vi "ProdaNG.Configurator.Popup.Add.vi"(6 "units simple":T1[](array[typedef]), 10 "Selected element":T2) -> (1 "Selected elements value out":T4, 2 "Selected element out":T2, 4 "Reason out":string, 5 "OK?":bool)   [LabVIEW 2016]
uses:
  ProdaNG.Tree.Fglb.Data.ctl
  ProdaNG.Tree.Fglb.Element.ctl
  ProdaNG.Tree.Fglb.Value.ctl
  Controls/ProdaNG.UnitSimple.ctl
panel:
  in  "Unit":i32(ring) items=["%"=1, "A"=12, "ASCII"=20, "Hz"=16, "N"=11, "Nm"=21, "V"=13, "angle"=17, "bar"=2, "bar (abs)"=3, "bar/s"=5, "bool"=19, "ccm/min"=24, "count"=18, "digit"=26, "kg"=22, "kohm"=15, "l/min"=7, "mA"=25, "mA/s"=30, "mBar/s"=29, "mbar"=4, "mbar/s"=6, "mm"=10, "ms"=9, "obr/min"=23, "ohm"=14, "s"=8, "stC"=28, "unknown"=-1, "us"=27]
  in  "Type":T5(ring)
  in  "Value2":dbl caption="High Limit" format="%.3f"
  in  "Value1":dbl caption="Low Limit / Param Value" format="%.3f"
  in  "Order":i32=1 min=1
  in  "Reason":string
  in  "Description":string
  in  "Button.Cancel":bool
  in  "Button.OK":bool
  out "Msg":string
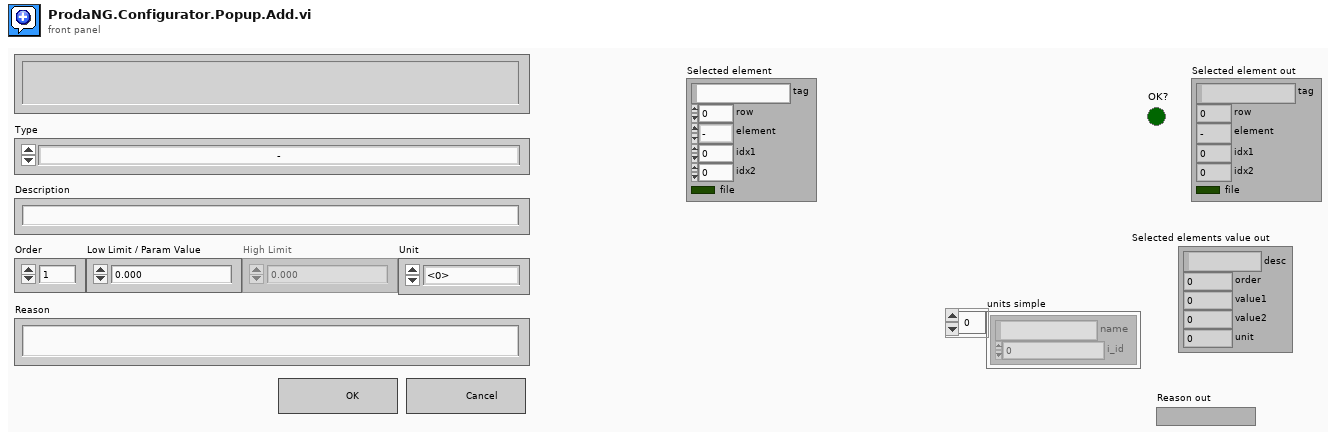
[diagram p1: front panel]
types:
  T1 = typedef "ProdaNG.UnitSimple.ctl" = cluster{"name":string, "i_id":i32}
  T2 = typedef "ProdaNG.Tree.Fglb.Data.ctl" = cluster{"tag":string, "row":i32, "element":T3, "idx1":i32, "idx2":i32, "file":bool}
  T3 = typedef "ProdaNG.Tree.Fglb.Element.ctl" = enum16{"-", "PP", "TS", "TP", "TV"}
  T4 = typedef "ProdaNG.Tree.Fglb.Value.ctl" = cluster{"desc":string, "order":i32, "value1":dbl, "value2":dbl, "unit":i32}
  T5 = enum16{"-", "Process Parameter", "Test Step", "Test Parameter", "Test Value"}
  T6 = enum8{"Enabled", "Disabled", "Disabled and Grayed Out"}
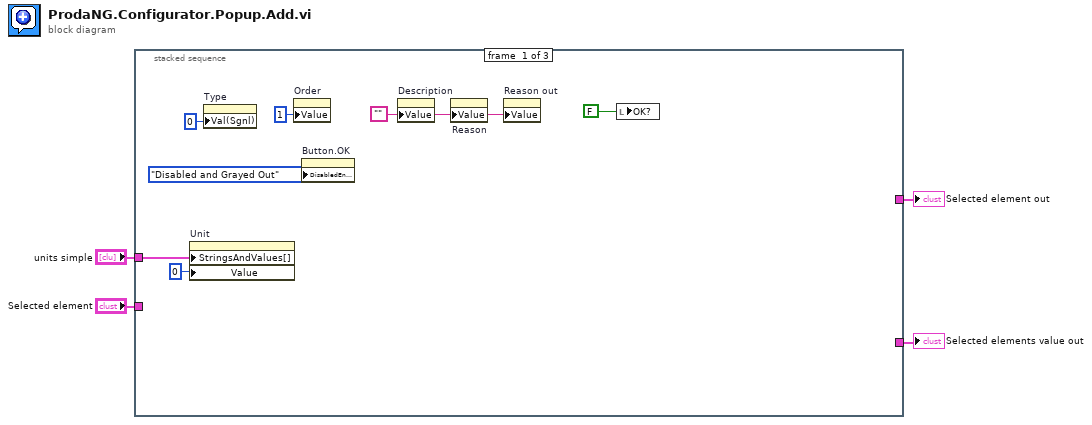
[diagram p0: block diagram]
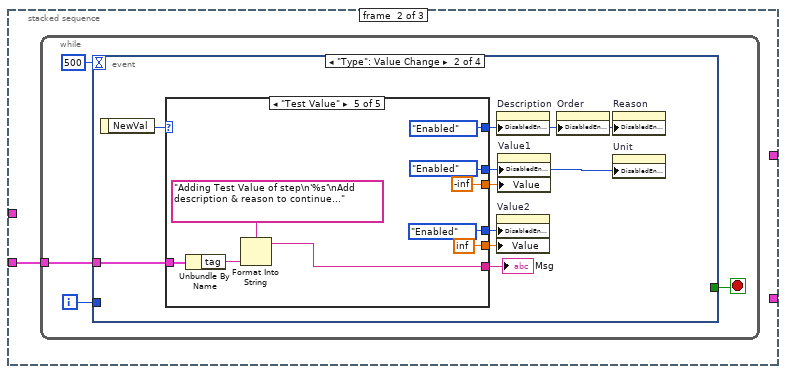
[diagram p2: hidden frame]
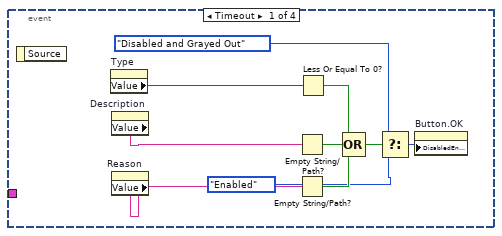
[diagram p3: hidden frame]
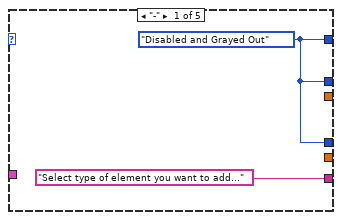
[diagram p4: hidden frame]
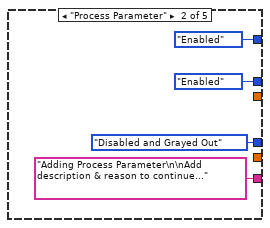
[diagram p5: hidden frame]
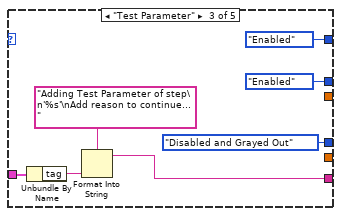
[diagram p6: hidden frame]
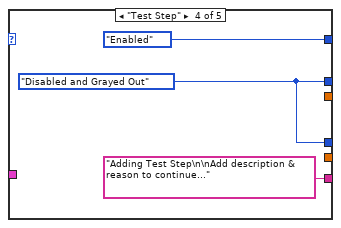
[diagram p7: hidden frame]
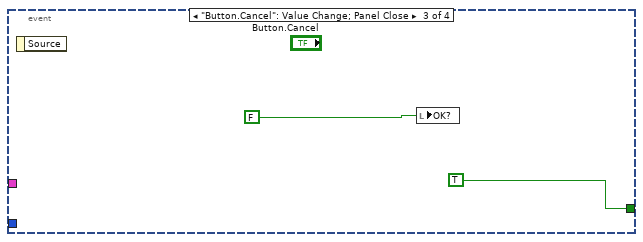
[diagram p8: hidden frame]
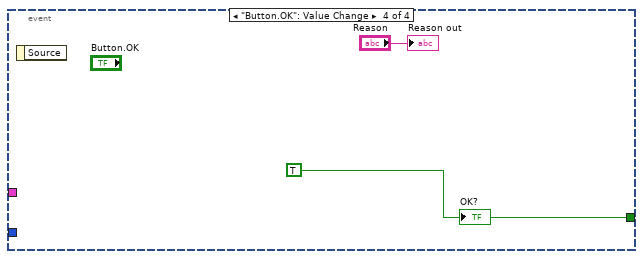
[diagram p9: hidden frame]
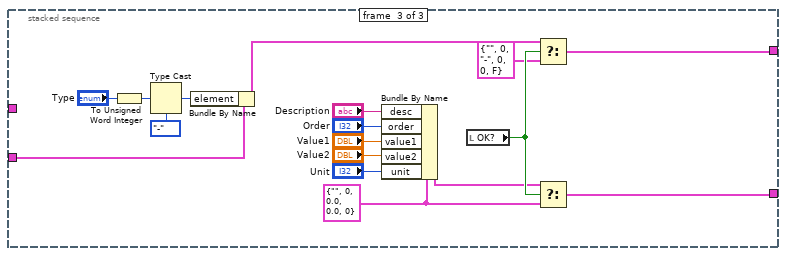
[diagram p10: hidden frame]
diagram:
  n1 = stacked-sequence {
    tunnel: [_ _ w80] -> w4
    tunnel: "Selected element" -> [_ w12 w78]
    tunnel: [_ _ w75] -> w2
    tunnel: "units simple" -> [w7 _ _]
    frame #0 {
      w9 = ""
      n2 = property on="Unit" class="Ring (strict)"("StringsAndValues[]"=w7, "Value"=0) -> ()  [unwired: 2 in, 2 out]
      n3 = property on="Type" class="Enum (strict)"("Val(Sgnl)"=0) -> ()  [unwired: 2 in, 2 out]
      n4 = property on="Order" class="DigNum (strict)"("Value"=1 ("Order")) -> ()  [unwired: 2 in, 2 out]
      n5 = property on="Button.OK" class="Bool"("DisabledEnum"=T6."Disabled and Grayed Out" ("Disabled")) -> ()  [unwired: 2 in, 2 out]
      n6 = property on="Description" class="Str"("Value"=w9) -> ()  [unwired: 2 in, 2 out]
      n7 = property on="Reason" class="Str"("Value"=w9) -> ()  [unwired: 2 in, 2 out]
      n8 = property on="Reason out" class="Str"("Value"=w9) -> ()  [unwired: 2 in, 2 out]
      n9 = local write "OK?"(FALSE ("OK?")) -> ()
    }
    frame #1 {
      n10 = while {
        tunnel: w12 -> [w13]
        i -> [w14]
        stop <- w16 stop-if-true
        n11 = event shown="[1] \"Type\": Value Change" {
          selector: _ -> [_ _ _ _]
          dyn-events: _ -> [_ _ _ _]
          timeout: 500 -> [_ _ _ _]
          tunnel: [_ _ TRUE ("OK?") w63] -> w16
          tunnel: w14 -> [_ _ _ _]
          tunnel: w13 -> [_ w29 _ _]
          event Timeout {
            n12 = event-data() -> ()  [unwired: 1 in, 1 out]
            n13 = property on="Type" class="Enum (strict)"() -> ("Value"=w22:T5)  [unwired: 2 in, 2 out]
            n14 = property on="Description" class="Str"() -> ("Value"=w20:string)  [unwired: 2 in, 2 out]
            n15 = property on="Reason" class="Str"() -> ("Value"=w21:string)  [unwired: 2 in, 2 out]
            n16 = Empty String/Path?(string/path=w20) -> (empty?=w23:bool)
            n17 = Empty String/Path?(string/path=w21) -> (empty?=w24:bool)
            n18 = Less Or Equal To 0?(x=w22) -> (x <= 0?=w25:bool)
            n19 = Compound Arithmetic op=OR(w25, w23, w24) -> (w26:bool)
            n20 = Select(t=T6."Disabled and Grayed Out" ("Disabled"), s=w26, f=T6."Enabled" ("Disabled")) -> (s? t:f=w17:T6)
            n21 = property on="Button.OK" class="Bool"("DisabledEnum"=w17) -> ()  [unwired: 2 in, 2 out]
          }
          event "Type": Value Change {
            n22 = event-data() -> ("NewVal"=w34:T5)  [unwired: 1 in]
            n23 = case shown="\"Test Value\"" w34 {
              tunnel: [w35 T6."Enabled" ("Disabled") T6."Enabled" ("Disabled") T6."Enabled" ("Disabled") T6."Enabled" ("Disabled")] -> w33
              tunnel: [w35 T6."Enabled" ("Disabled") T6."Enabled" ("Disabled") w49 T6."Enabled" ("Disabled")] -> w30
              tunnel: [_ _ _ _ -inf] -> w32
              tunnel: [_ _ _ _ inf] -> w31
              tunnel: w29 -> [_ _ w42 _ w54]
              tunnel: ["Select type of element you want to add..." ("format string") "Adding Process Parameter\n\nAdd description & reason to continue..." ("format string") w41 "Adding Test Step\n\nAdd description & reason to continue..." ("format string") w51] -> w28
              tunnel: [w35 T6."Disabled and Grayed Out" ("Disabled") T6."Disabled and Grayed Out" ("Disabled") w49 T6."Enabled" ("Disabled")] -> w27
              frame "-" {
                w35 = T6."Disabled and Grayed Out" ("Disabled")
              }
              frame "Process Parameter" {
              }
              frame "Test Parameter" {
                n24 = Unbundle By Name(w42) -> ("tag"=w44:string)
                n25 = Format Into String(format string="Adding Test Parameter of step\n'%s'\nAdd reason to continue...", w44) -> (resulting string=w41:string)  [unwired: 2 in, 1 out]
              }
              frame "Test Step" {
                w49 = T6."Disabled and Grayed Out" ("Disabled")
              }
              frame "Test Value" {
                n26 = Unbundle By Name(w54) -> ("tag"=w53:string)
                n27 = Format Into String(format string="Adding Test Value of step\n'%s'\nAdd description & reason to continue...", w53) -> (resulting string=w51:string)  [unwired: 2 in, 1 out]
              }
            }
            "Msg" <- w28
            n28 = property on="Description" class="Str"("DisabledEnum"=w33) -> ()  [unwired: 2 in, 2 out]
            n29 = property on="Value2" class="DigNum (strict)"("DisabledEnum"=w27, "Value"=w31) -> ()  [unwired: 2 in, 2 out]
            n30 = property on="Value1" class="DigNum (strict)"("DisabledEnum"=w30, "Value"=w32) -> ()  [unwired: 2 in, 2 out]
            n31 = property on="Order" class="DigNum (strict)"("DisabledEnum"=w33) -> ()  [unwired: 2 in, 2 out]
            n32 = property on="Reason" class="Str"("DisabledEnum"=w33) -> ()  [unwired: 2 in, 2 out]
            n33 = property on="Unit" class="Ring (strict)"("DisabledEnum"=w30) -> ()  [unwired: 2 in, 2 out]
          }
          event "Button.Cancel": Value Change; Panel Close {
            n34 = event-data() -> ()  [unwired: 1 in, 1 out]
            n35 = local write "OK?"(FALSE ("OK?")) -> ()
          }
          event "Button.OK": Value Change {
            w63 = TRUE ("OK?")
            n36 = event-data() -> ()  [unwired: 1 in, 1 out]
            "OK?" <- w63
            "Reason out" <- "Reason"
          }
        }
      }
    }
    frame #2 {
      w64 = T4 {"desc"="", "order"=0, "value1"=0.0, "value2"=0.0, "unit"=0} ("Value")
      n37 = To Unsigned Word Integer(number="Type") -> (unsigned 16bit integer=w72:u16)
      n38 = Type Cast(type=ProdaNG.Tree.Fglb.Element."-" ("element"), x=w72) -> (*(type *) &x=w73:T3)
      n39 = Bundle By Name(cluster=w78, "element"=w73) -> (w77:T2)
      n40 = Bundle By Name(cluster=w64, "desc"="Description", "order"="Order", "value1"="Value1", "value2"="Value2", "unit"="Unit") -> (w66:T4)
      n41 = local read "OK?"() -> (w79:bool)
      n42 = Select(t=w77, s=w79, f=T2 {"tag"="", "row"=0, "element"=enum."-", "idx1"=0, "idx2"=0, "file"=FALSE}) -> (s? t:f=w75:T2)
      n43 = Select(t=w66, s=w79, f=w64) -> (s? t:f=w80:T4)
    }
  }
  "Selected elements value out" <- w4
  "Selected element out" <- w2
